vi "Send Channel Settings.vi"(6 "Value to Send":T1, 8 "error in":errorcluster, 10 "Channel List":T2, 11 "SimELoad in":refnum<class "SimEload.lvclass">) -> (0 "error out":errorcluster, 3 "SimELoad out":refnum<class "SimEload.lvclass">)   [LabVIEW 2019, in "SimELoad.lvlib" / "SimEload.lvclass"]
uses:
  SimEload.lvclass
  builds/Instruments/Electronic Load.lvlibp/Custom Controls/Channel Select.ctl
  C:/Users/Public/Documents/Development/builds/Instruments/Electronic Load.lvlibp/Electronic Load.lvclass
  builds/Instruments/Electronic Load.lvlibp/Custom Controls/Value to Send.ctl
  Accessors/Read Local Resource.vi
  builds/Instruments/Electronic Load.lvlibp/Accessors/Read Function Array.vi
  builds/Instruments/Electronic Load.lvlibp/Electronic Load.lvclass
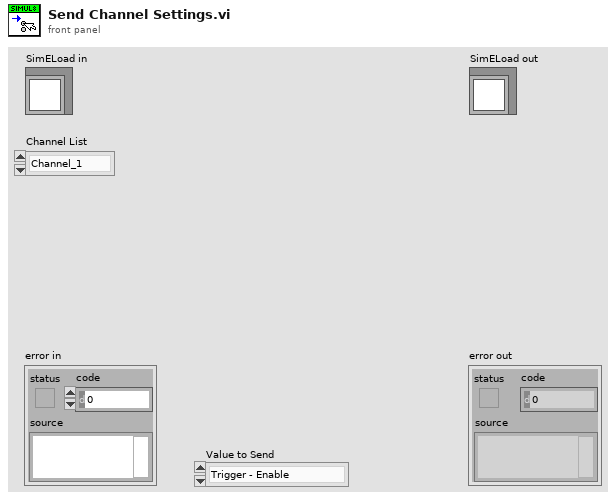
[diagram p1: front panel]
types:
  T1 = typedef "Electronic Load.lvlibp/Electronic Load.lvclass/Value to Send.ctl" = enum16{"Trigger - Enable", "Trigger - Sample Interval", "Trigger - Data Points", "Trigger - Current(Initial)", "Trigger - Transient Current", "Trigger - Pulse Width", "Trigger - Delay", "OCP - Enable", "OCP - Level", "OCP - Delay", "Function - Mode", "Function - Value", "Function - Enabled"}
  T2 = typedef "Electronic Load.lvlibp/Electronic Load.lvclass/Channel Select.ctl" = enum16{"Channel_1", "Channel_2", "Channel_3", "Channel_4", "Channel_5", "Channel_6"}
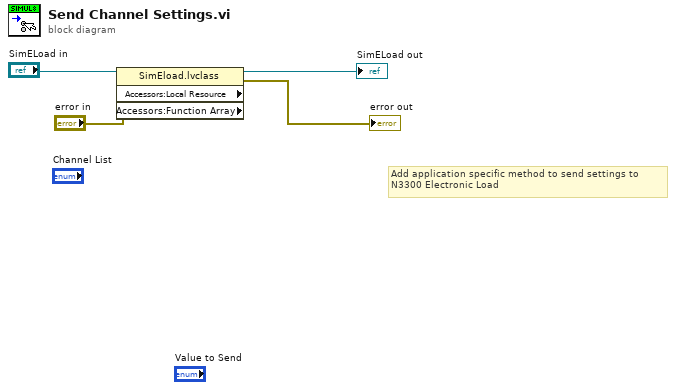
[diagram p0: block diagram]
diagram:
  # "Add application specific method to send settings to \nN3300 Electronic Load"
  n1 = property class="SimEload.lvclass" props=["Accessors:Local Resource", "Accessors:Function Array"](reference="SimELoad in", error in="error in") -> (reference out=→"SimELoad out":refnum<class "SimEload.lvclass">, error out=→"error out":errorcluster)  [unwired: 2 out]
